vi "NML VISA Send Multiple Commands.vi"(8 "error in (no error)":errorcluster, 10 "Commands":string[](array[string]), 11 "VISA resource name":refnum<visa-resource-name>) -> (3 "VISA resource name":refnum<visa-resource-name>)   [LabVIEW 2025]
doc: "VI to send (no readback) multiple commands over VISA. VISA ref will be opened if necessary\n\nScott Hannahs <sth@magnet.fsu.edu> May 2022\nAuthor: Scott Hannahs <sth@magnet.fsu.edu>\n\nThis software is licensed for use under the “MIT License\"\nCopyright (c) 2025 Scott Hannahs, sth@sth@magnet.sthnet.net\n\nPermission is hereby granted, free of charge, to any person obtaining a copy of this software and associated documentation files (the \"Software\"), to deal in the Software without restriction, including without limitation the rights to use, copy, modify, merge, publish, distribute, sublicense, and/or sell copies of the Software, and to permit persons to whom the Software is furnished to do so, subject to the following conditions: The above copyright notice and this permission notice shall be included in all copies or substantial portions of the Software.\n\nTHE SOFTWARE IS PROVIDED \"AS IS\", WITHOUT WARRANTY OF ANY KIND, EXPRESS OR IMPLIED, INCLUDING BUT NOT LIMITED TO THE WARRANTIES OF MERCHANTABILITY, FITNESS FOR A PARTICULAR PURPOSE AND NONINFRINGEMENT. IN NO EVENT SHALL THE AUTHORS OR COPYRIGHT HOLDERS BE LIABLE FOR ANY CLAIM, DAMAGES OR OTHER LIABILITY, WHETHER IN AN ACTION OF CONTRACT, TORT OR OTHERWISE, ARISING FROM, OUT OF OR IN CONNECTION WITH THE SOFTWARE OR THE USE OR OTHER DEALINGS IN THE SOFTWARE."
panel:
  out "error out":errorcluster
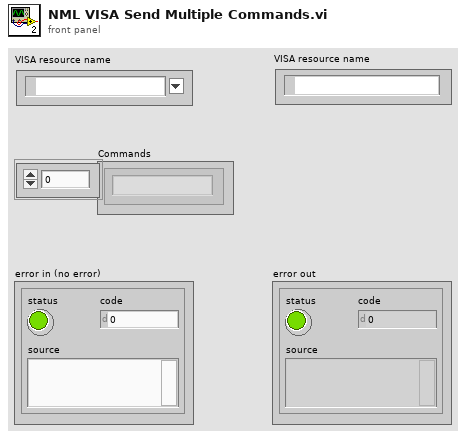
[diagram p1: front panel]
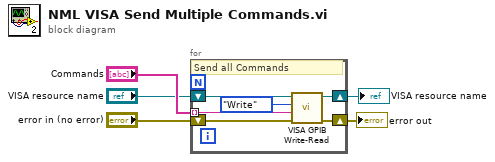
[diagram p0: block diagram]
diagram:
  n1 = for {
    shift-right: [w10] -> w3
    shift-left: "VISA resource name" -> [w11]
    tunnel: "Commands" -> [w8] mode=indexing
    shift-right: [w6] -> w1
    shift-left: "error in (no error)" -> [w7]
    # "Send all Commands"
    n2 = call "VISA GPIB Write-Read.vi"("error in (no error)"=w7, "Command"=w8, "Action"=enum16{"Write", "Read", "Write & Read"}."Write", "VISA resource name"=w11) -> ("error out"=w6:errorcluster, "dup VISA Session"=w10:refnum<visa-resource-name>)  [unwired: 4 in, 2 out]
  }
  "VISA resource name" <- w3
  "error out" <- w1
